vi "Equal - Boolean.vi"(0 "Value In":bool) -> (4 "Previous Value":bool, 15 "Equal to previous value":bool)   [LabVIEW 2011]
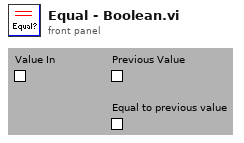
[diagram p1: front panel]
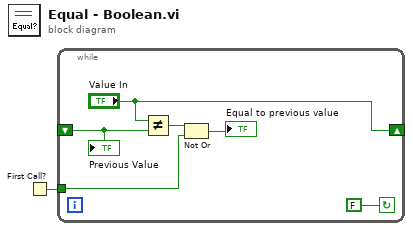
[diagram p0: block diagram]
diagram:
  n1 = First Call?() -> (First Call?: T/F=w1:bool)
  n2 = while {
    tunnel: w1 -> [w4]
    shift-right: ["Value In"] -> _
    shift-left: _ -> [w3]
    stop <- FALSE continue-if-true
    n3 = Not Equal?(x="Value In", y=w3) -> (x != y?=w5:bool)
    n4 = Not Or(1:w4, 2:w5) -> (0:→"Equal to previous value":bool)
    "Previous Value" <- w3
  }
